vi "Test PWM Output.vi"(8 "error in":errorcluster, 10 "TestCase in":refnum<class "Scan Engine Scripting API Modules.lvclass">, 11 "module test in":refnum<class "Module Test.lvclass">) -> (0 "error out":errorcluster, 2 "TestCase out":refnum<class "Scan Engine Scripting API Modules.lvclass">, 3 "module test out":refnum<class "Module Test.lvclass">)   [LabVIEW 2019, in "Module Test.lvclass"]
uses:
  Module Test.lvclass
  Scan Engine Scripting API Modules.lvclass
  C:/Program Files (x86)/National Instruments/LabVIEW 2019/vi.lib/addons/_JKI Toolkits/VI Tester/TestCase.llb/TestCase.lvclass
  Scripting/Modules/Mode Classes/Controls/pwm channel settings.ctl
  Scripting/Modules/Channel Classes/PWM Output Channel/Frequency.ctl
  Module Test.lvclass/Module Test.ctl
  Scripting/Modules/Channel Classes/PWM Output Channel/PWM Output Channel.lvclass
  Scripting/Scan Engine Scripting.lvlib
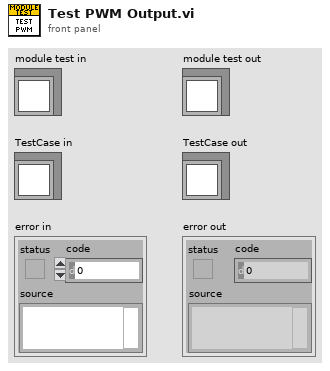
[diagram p1: front panel]
types:
  T1 = typedef "Scan Engine Scripting.lvlib/pwm channel settings.ctl" = cluster{"name":string, "default value":dbl, "frequency":T2}
  T2 = typedef "Scan Engine Scripting.lvlib/PWM Output Channel.lvclass/Frequency.ctl" = enum16{"1 Hz (1,000,000 us)", "50 Hz (20,000 us)", "250 Hz (4,000 us)", "500 Hz (2,000 us)", "1 kHz (1,000 us)", "5 kHz (200 us)", "10 kHz (100 us)", "20 kHz (50 us)"}
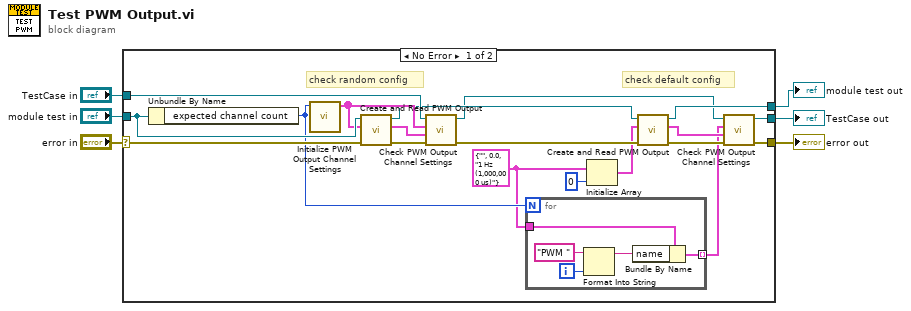
[diagram p0: block diagram]
diagram:
  n1 = case shown="No Error" "error in" {
    selector: "error in" -> [w25 w33]
    tunnel: [w12 w33] -> w5
    tunnel: [w17 w32] -> w3
    tunnel: "module test in" -> [w24 w32]
    tunnel: "TestCase in" -> [w23 w31]
    tunnel: [w13 w31] -> w1
    frame No Error {
      w9 = T1 {"name"="", "default value"=0.0, "frequency"=enum."1 Hz (1,000,000 us)"} ("channel settings")
      # "check default config"
      # "check random config"
      n2 = Unbundle By Name(w24) -> ("expected channel count"=w11:i32)
      n3 = call "Initialize PWM Output Channel Settings.vi"("array size"=w11) -> ("channel settings"=w21:T1[])  [unwired: 10 in]
      n4 = call-dynamic "Create and Read PWM Output.vi"("error in"=w25, "channel settings in"=w21, "module test in"=w24) -> ("error out"=w22:errorcluster, "channel settings out"=w20:T1[], "module test out"=w18:refnum<class "Module Test.lvclass">)  [unwired: 6 in]
      n5 = call "Check PWM Output Channel Settings.vi"("error in"=w22, "read channel settings"=w20, "initial channel settings"=w21, "TestCase in"=w23) -> ("error out"=w19:errorcluster, "TestCase out"=w14:refnum<class "Scan Engine Scripting API Modules.lvclass">)  [unwired: 6 in]
      n6 = for {
        N: w11 -> [_]
        tunnel: [w27] -> w10 mode=indexing
        tunnel: w9 -> [w26]
        i -> [w30]
        n7 = Format Into String(initial string="PWM ", w30) -> (resulting string=w28:string)  [unwired: 2 in, 1 out]
        n8 = Bundle By Name(cluster=w26, "name"=w28) -> (w27:T1)
      }
      n9 = Initialize Array(w9, 0 ("dimension size")) -> (w8:T1[])
      n10 = call-dynamic "Create and Read PWM Output.vi"("error in"=w19, "channel settings in"=w8, "module test in"=w18) -> ("error out"=w15:errorcluster, "channel settings out"=w16:T1[], "module test out"=w17:refnum<class "Module Test.lvclass">)  [unwired: 6 in]
      n11 = call "Check PWM Output Channel Settings.vi"("error in"=w15, "read channel settings"=w16, "initial channel settings"=w10, "TestCase in"=w14) -> ("error out"=w12:errorcluster, "TestCase out"=w13:refnum<class "Scan Engine Scripting API Modules.lvclass">)  [unwired: 6 in]
    }
    frame Error {
    }
  }
  "error out" <- w5
  "module test out" <- w3
  "TestCase out" <- w1
